vi "Show symbols Write.vi"(4 "error in (no error)":errorcluster, 5 "Value":bool, 6 "Container State":T2, 7 "Display State In":T1) -> (0 "error out":errorcluster, 3 "Display State Out":T1)   [LabVIEW 2020, in "KLegend.xctl"]
uses:
  KLegend.xctl
  <vilib>/_xctls/Container State.ctl
  <vilib>/_xctls/XControlSupport.lvlib
  State.vi
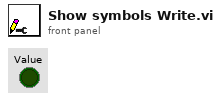
[diagram p1: front panel]
types:
  T1 = typedef "KLegend.xctl/State.vi" = cluster{"Plot":refnum<vi>, "Vals":dbl[], "fmt":string, "cmd":string, "max rows":i32, "show symbols":bool}
  T2 = typedef "XControlSupport.lvlib/Container State.ctl" = cluster{"Indicator?":bool, "Run Mode?":bool, " Refnum":refnum<vi>}
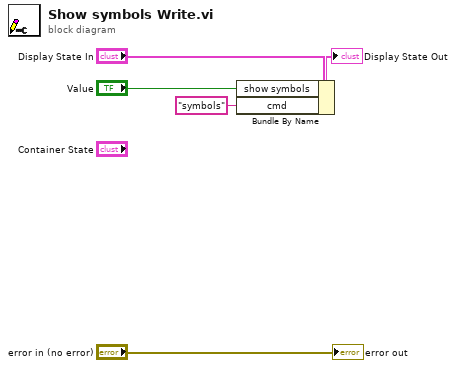
[diagram p0: block diagram]
diagram:
  n1 = Bundle By Name(cluster="Display State In", "show symbols"="Value", "cmd"="symbols") -> (→"Display State Out":T1)
  "error out" <- "error in (no error)"
